vi "get_TLC_type.vi"(8 "error in (no error)":errorcluster, 11 "GenericToplevelComponent in":refnum<class "GenericToplevelComponent.lvclass">) -> (0 "error out":errorcluster, 2 "top-level component type":T1, 3 "GenericToplevelComponent out":refnum<class "GenericToplevelComponent.lvclass">)   [LabVIEW 2010, in "GenericToplevelComponent.lvclass"]
uses:
  GenericToplevelComponent.lvclass
  enumerations/top-level_component_type_enum.ctl
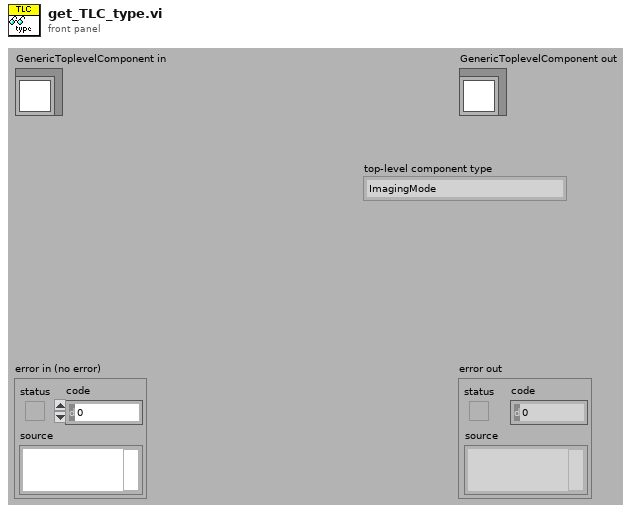
[diagram p1: front panel]
types:
  T1 = typedef "top-level_component_type_enum.ctl" = enum16{"ImagingMode", "ScanHead", "DAQ", "ImageAssembler", "Display", "DataCollection", "Analyser", "Stimulator", "ExperimentController", "Instrument", "Stage"}
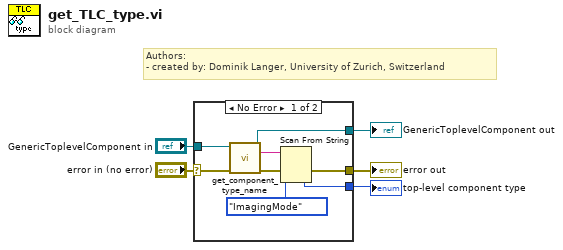
[diagram p0: block diagram]
diagram:
  # "Authors: \n- created by: Dominik Langer, University of Zurich, Switzerland"
  n1 = case shown="No Error" "error in (no error)" {
    selector: "error in (no error)" -> [w13 w15]
    tunnel: [w10 w15] -> w4
    tunnel: [w8 w14] -> w2
    tunnel: "GenericToplevelComponent in" -> [w9 w14]
    tunnel: [w7 _] -> w1
    frame No Error {
      n2 = call-dynamic "get_component_type_name.vi"("error in (no error)"=w13, "GenericPlugin in"=w9) -> ("error out"=w11:errorcluster, "component type"=w6:string, "GenericPlugin out"=w8:refnum<class "GenericToplevelComponent.lvclass">)  [unwired: 7 in]
      n3 = Scan From String(input string=w6, error in=w11, default 1=top-level_component_type_enum."ImagingMode" ("top-level component type 2")) -> (error out=w10:errorcluster, output 1=w7:T1)  [unwired: 2 in, 2 out]
    }
    frame Error {
    }
  }
  "error out" <- w4
  "GenericToplevelComponent out" <- w2
  "top-level component type" <- w1
